vi "Read Coils.vi"(8 "error in":errorcluster, 9 "number of coils":u16, 10 "starting address":u16, 11 "device data model in":refnum<class "Standard Data Model.lvclass">) -> (0 "error out":errorcluster, 2 "data":bool[](array[boolean]), 3 "device data model out":refnum<class "Standard Data Model.lvclass">)   [LabVIEW 2012, in "Standard Data Model.lvclass"]
doc: "Reads N coils from the data model starting at address M."
uses:
  Standard Data Model.lvclass
  Standard Data Model.lvclass/Standard Data Model.ctl
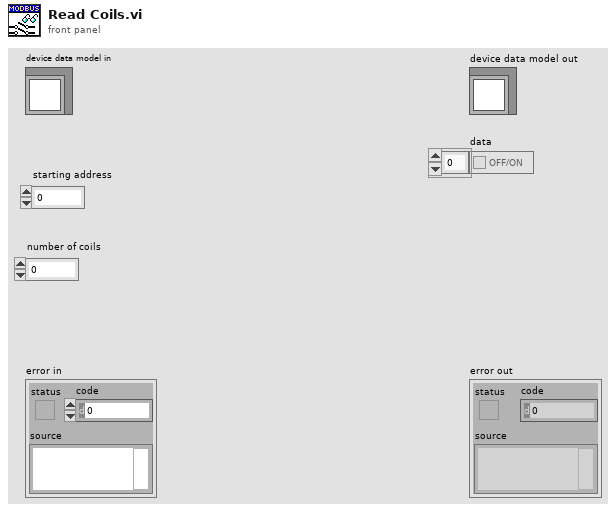
[diagram p1: front panel]
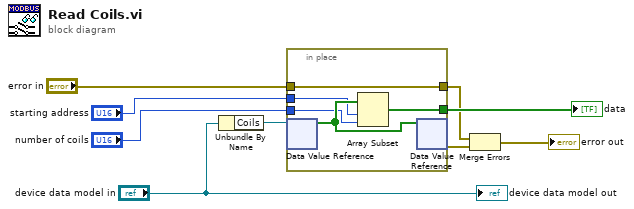
[diagram p0: block diagram]
diagram:
  n1 = Unbundle By Name("device data model in") -> ("Coils"=w6:refnum<data-value>)
  n2 = in-place {
    in-place-border: "error in" -> [w14]
    in-place-border: [w14] -> w3
    in-place-border: [w12] -> w5
    in-place-border: "starting address" -> [w11]
    in-place-border: "number of coils" -> [w10]
    n3 = in-place-dvr #1(w6) -> (w13:bool[])  [unwired: 1 out]
    n4 = Array Subset(array=w13, index=w11, length=w10) -> (w12:bool[])
    n5 = in-place-dvr #1(w13) -> (w4:errorcluster)  [unwired: 1 out]
  }
  "data" <- w5
  n6 = Merge Errors(w3, w4) -> (→"error out":errorcluster)
  "device data model out" <- "device data model in"
